vi "AddBandstoBandNames.vi"(11 "filter name":string) -> (1 "File Name":string[](array[string]), 3 "Extended Name":string[](array[string]))   [LabVIEW 2022 SP3]
uses:
  <vilib>/Utility/error.llb/whitespace.ctl
  <vilib>/Utility/error.llb/Trim Whitespace One-Sided.vi
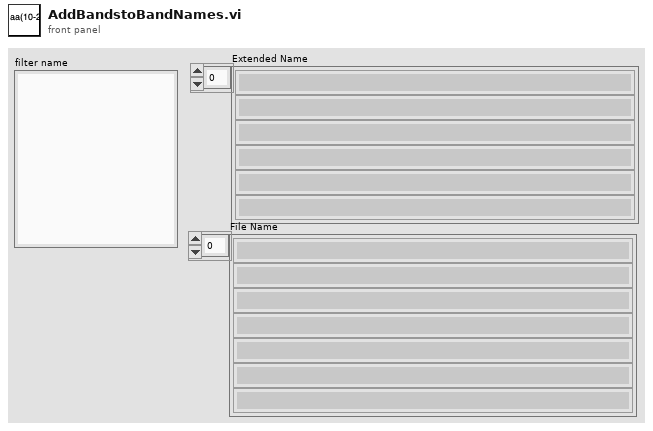
[diagram p1: front panel]
types:
  T1 = typedef "whitespace.ctl" = u16
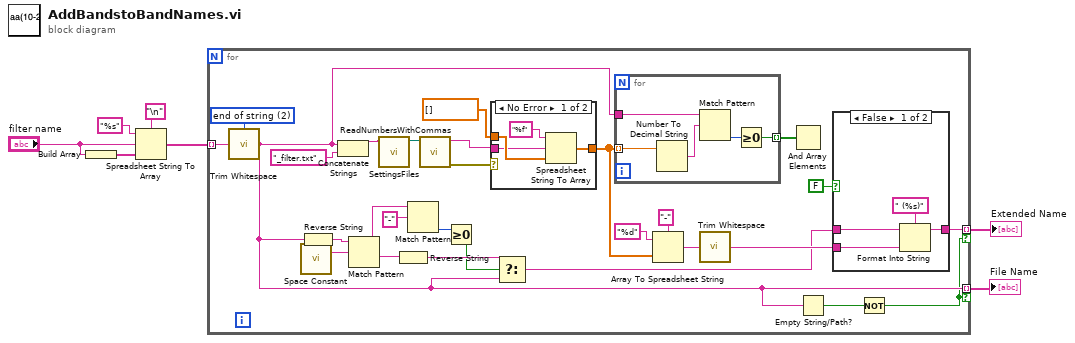
[diagram p0: block diagram]
diagram:
  n1 = Build Array("filter name") -> (w5:string[])
  n2 = Spreadsheet String To Array(delimiter (Tab)="\n" ("format string"), format string="%s", spreadsheet string="filter name", array type (2D Dbl)=w5) -> (array=w4:string[])
  n3 = for {
    tunnel: w4 -> [w25] mode=indexing
    tunnel: [w29] -> w3 mode=indexing if=w14
    tunnel: [w16] -> w2 mode=indexing if=w14
    w11 = T1 2 items=["both", "start of string", "end of string"] ("location (both)")
    n4 = call <vilib>:"Trim Whitespace.vi"("string"=w25, "location (both)"=w11) -> ("trimmed string"=w16:string)
    n5 = call <vilib>:"Space Constant.vi"() -> ("String"=w23:string)
    n6 = Reverse String(1:w16) -> (0:w24:string)
    n7 = Concatenate Strings(w16, "_filter.txt" ("string")) -> (w35:string)
    n8 = Match Pattern(string=w24, regular expression=w23) -> (before substring=w13:string, after substring=w22:string)  [unwired: 1 in, 2 out]
    n9 = call "SettingsFiles.vi"("settings file name"=w35) -> ("file path"=w9:path)  [unwired: 9 in, 1 out]
    n10 = Reverse String(1:w22) -> (0:w20:string)
    n11 = Match Pattern(string=w13, regular expression="-" ("delimiter (Tab)")) -> (offset past match=w18:i32)  [unwired: 1 in, 3 out]
    n12 = call "ReadNumbersWithCommas.vi"("file (use dialog)"=w9) -> ("error out"=w10:errorcluster, "fixed"=w8:string)  [unwired: 7 in, 2 out]
    n13 = Greater Or Equal To 0?(x=w18) -> (x >= 0?=w17:bool)
    n14 = case shown="No Error" w10 {
      tunnel: [w47 w50] -> w26
      tunnel: w8 -> [w46 _]
      tunnel: dbl[] [] ("DataPath") -> [w49 w50]
      frame No Error {
        n15 = Spreadsheet String To Array(format string="%f", spreadsheet string=w46, array type (2D Dbl)=w49) -> (array=w47:dbl[])  [unwired: 1 in]
      }
      frame Error {
      }
    }
    n16 = Select(t=w20, s=w17, f=w16) -> (s? t:f=w19:string)
    n17 = for {
      tunnel: [w36] -> w28 mode=indexing
      tunnel: w16 -> [w39]
      tunnel: w26 -> [w38] mode=indexing
      n18 = Number To Decimal String(number=w38) -> (decimal integer string=w37:string)  [unwired: 1 in]
      n19 = Match Pattern(string=w39, regular expression=w37) -> (offset past match=w40:i32)  [unwired: 1 in, 3 out]
      n20 = Greater Or Equal To 0?(x=w40) -> (x >= 0?=w36:bool)
    }
    n21 = Array To Spreadsheet String(delimiter (Tab)="-", array=w26, 3:"%d" ("format string")) -> (spreadsheet string=w30:string)
    n22 = call <vilib>:"Trim Whitespace.vi"("string"=w30) -> ("trimmed string"=w27:string)  [unwired: 1 in]
    n23 = And Array Elements(Boolean array=w28) -> ()  [unwired: 1 out]
    n24 = Empty String/Path?(string/path=w16) -> (empty?=w15:bool)
    n25 = case shown="False" FALSE {
      tunnel: w19 -> [w43 w45]
      tunnel: [w42 w45] -> w29
      tunnel: w27 -> [w41 _]
      frame False {
        n26 = Format Into String(format string=" (%s)", initial string=w43, w41) -> (resulting string=w42:string)  [unwired: 1 in, 1 out]
      }
      frame True {
      }
    }
    n27 = Not(x=w15) -> (.not. x?=w14:bool)
  }
  "Extended Name" <- w3
  "File Name" <- w2
